vi "Print List of Hardware (DevInfo).vi"(9 "Devices":refnum<class "DevInfo.lvclass">[](array[class])) -> (3 "String":string)   [LabVIEW 2016, in "Controller Actor.lvlib" / "Controller.lvclass"]
uses:
  <userlib>/Common Components/Controller/Controller.lvclass
  <userlib>/Common Components/Hardware/DevInfo/DevInfo.lvclass
  <userlib>/Common Components/Hardware/DevInfo/DevInfo.lvclass/DevInfo.ctl
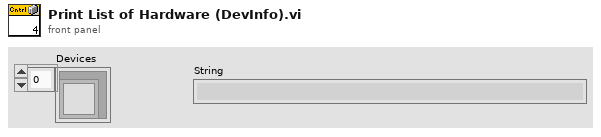
[diagram p1: front panel]
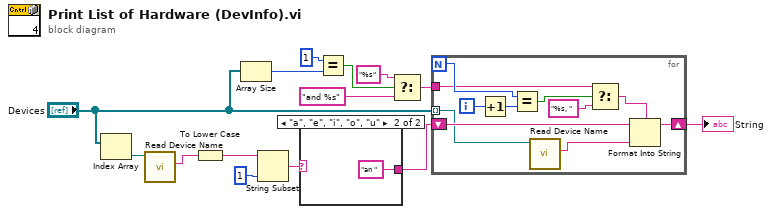
[diagram p0: block diagram]
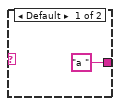
[diagram p2: hidden frame]
diagram:
  n1 = Index Array(array="Devices") -> (element=w6:refnum<class "DevInfo.lvclass">)  [unwired: 1 in]
  n2 = call <userlib>:"Read Device Name.vi"("DevInfo in"=w6) -> ("Device Name"=w1:string)  [unwired: 8 in, 2 out]
  n3 = To Lower Case(string=w1) -> (all lower case string=w5:string)
  n4 = Array Size(array="Devices") -> (size(s)=w13:i32)
  n5 = String Subset(string=w5, length (rest)=1 ("length (rest)")) -> (substring=w3:string)  [unwired: 1 in]
  n6 = case shown="\"a\", \"e\", \"i\", \"o\", \"u\"" w3 {
    tunnel: ["a " "an "] -> w2
    frame Default {
    }
    frame "a", "e", "i", "o", "u" {
    }
  }
  n7 = Equal?(x=1, y=w13) -> (x = y?=w11:bool)
  n8 = Select(t="%s", s=w11, f="and %s" ("format string")) -> (s? t:f=w9:string)
  n9 = for {
    N -> [w22]
    shift-right: [w27] -> w14
    shift-left: w2 -> [w26]
    tunnel: "Devices" -> [w25] mode=indexing
    tunnel: w9 -> [w18]
    i -> [w24]
    n10 = Increment(x=w24) -> (x+1=w23:i32)
    n11 = Equal?(x=w22, y=w23) -> (x = y?=w21:bool)
    n12 = call <userlib>:"Read Device Name.vi"("DevInfo in"=w25) -> ("Device Name"=w17:string)  [unwired: 8 in, 2 out]
    n13 = Select(t=w18, s=w21, f="%s, " ("format string")) -> (s? t:f=w19:string)
    n14 = Format Into String(format string=w19, initial string=w26, w17) -> (resulting string=w27:string)  [unwired: 1 in, 1 out]
  }
  "String" <- w14
